vi "Send Batch.vi"(8 "error in (no error)":errorcluster, 9 "Message Priority (Normal)":T1=enum."Normal", 10 "Messages Array":refnum<class "Message.lvclass">[](array[class]), 11 "Message Enqueuer":refnum<class "Message Enqueuer.lvclass">) -> (0 "error out":errorcluster)   [LabVIEW 2020, in "AF Specialty Messages.lvlib" / "Batch Msg.lvclass"]
doc: "<p>(<strong>Filename</strong>: <span class=\"dnl\">Actor Framework.lvlib:Batch Msg.lvclass:Send Batch.vi</span>)</p>\n\n<p>Sends multiple messages in a batch to an actor. All messages in the batch are given the same priority. No additional messages of the same priority will be processed by the actor in between the messages in the batch. However, messages with a higher priority than the batch will be processed before the batch itself.</p>"
uses:
  Batch Msg.lvclass
  Message/Message.lvclass
  Message Enqueuer/Message Enqueuer.lvclass
  Batch Msg.lvclass/Batch Msg.ctl
  Message Enqueuer/Message Priority.ctl
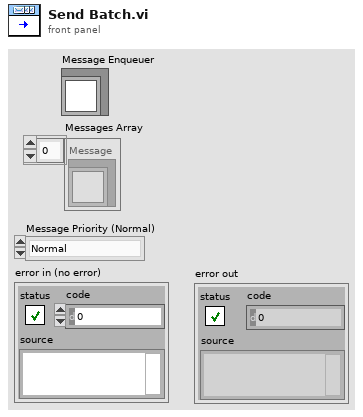
[diagram p1: front panel]
types:
  T1 = typedef "Actor Framework.lvlib/Message Enqueuer.lvclass/Message Priority.ctl" = enum16{"Low", "Normal", "High"}
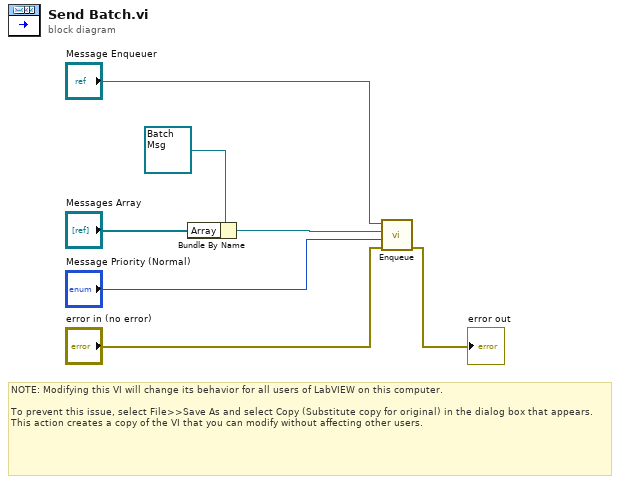
[diagram p0: block diagram]
diagram:
  # "NOTE: Modifying this VI will change its behavior for all users of LabVIEW on this computer.\n\nTo prevent this issue, select File>>Save As and select Copy (Substitute copy for original) in the dialog box that appears. This action creates a copy of the VI that you can modify without affecting other users."
  n1 = Bundle By Name(cluster=refnum<class "Batch Msg.lvclass"> refnum ("Batch Message.lvclass"), "Array"="Messages Array") -> (w2:refnum<class "Batch Msg.lvclass">)
  n2 = call "Enqueue.vi"("error in (no error)"="error in (no error)", "Message Priority (Normal)"="Message Priority (Normal)", "Message"=w2, "Message Enqueuer in"="Message Enqueuer") -> ("error out"=→"error out":errorcluster)  [unwired: 6 in, 1 out]
